vi "GenerateIncrementalBuildInfo.vi"(8 "error in (no error)":errorcluster, 9 "Generated file":T1, 11 "SolutionBuilder in":refnum<class "SolutionBuilder.lvclass">) -> (0 "error out":errorcluster, 3 "SolutionBuilder out":refnum<class "SolutionBuilder.lvclass">)   [LabVIEW 2019, in "SolutionBuilder.lvlib" / "SolutionBuilder.lvclass"]
uses:
  SolutionBuilder.lvclass
  BuildManager/GeneratedFile.ctl
  SolutionBuilder.lvclass/SolutionBuilder.ctl
  Private/IncrementalFileInfoHash.ctl
  Community/SolutionProjectInfo.ctl
  BuildManager/BuildManager.lvclass
  BuildManager/BuildProjectInfo.ctl
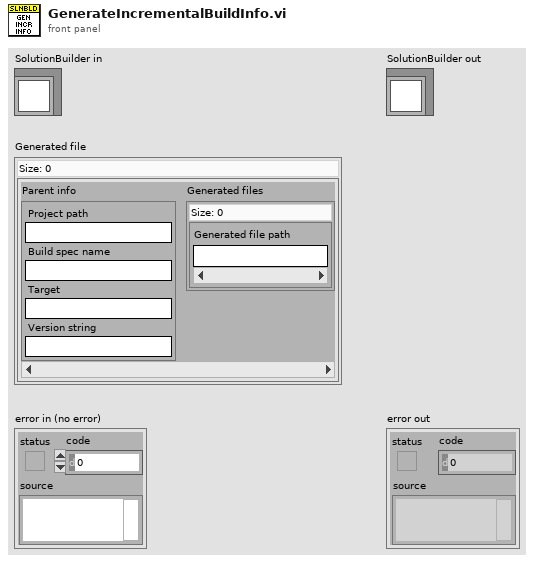
[diagram p1: front panel]
types:
  T1 = typedef "SolutionBuilder.lvlib/BuildManager.lvclass/GeneratedFile.ctl" = map{T2, set{string}}
  T2 = typedef "SolutionBuilder.lvlib/BuildManager.lvclass/BuildProjectInfo.ctl" = cluster{"Project path":string, "Build spec name":string, "Target":string, "Version string":string}
  T3 = typedef "SolutionBuilder.lvlib/SolutionBuilder.lvclass/HashMap.ctl" = map{T4, map{string, string}}
  T4 = typedef "SolutionBuilder.lvlib/SolutionBuilder.lvclass/SolutionProjectInfo.ctl" = cluster{"Project path":string, "Build spec name":string, "Target":string}
  T5 = typedef "SolutionBuilder.lvlib/SolutionBuilder.lvclass/IncrementalFileInfoHash.ctl" = cluster{"Project path":string, "Build spec name":string, "Target":string, "File":string, "MD5 hash":string}
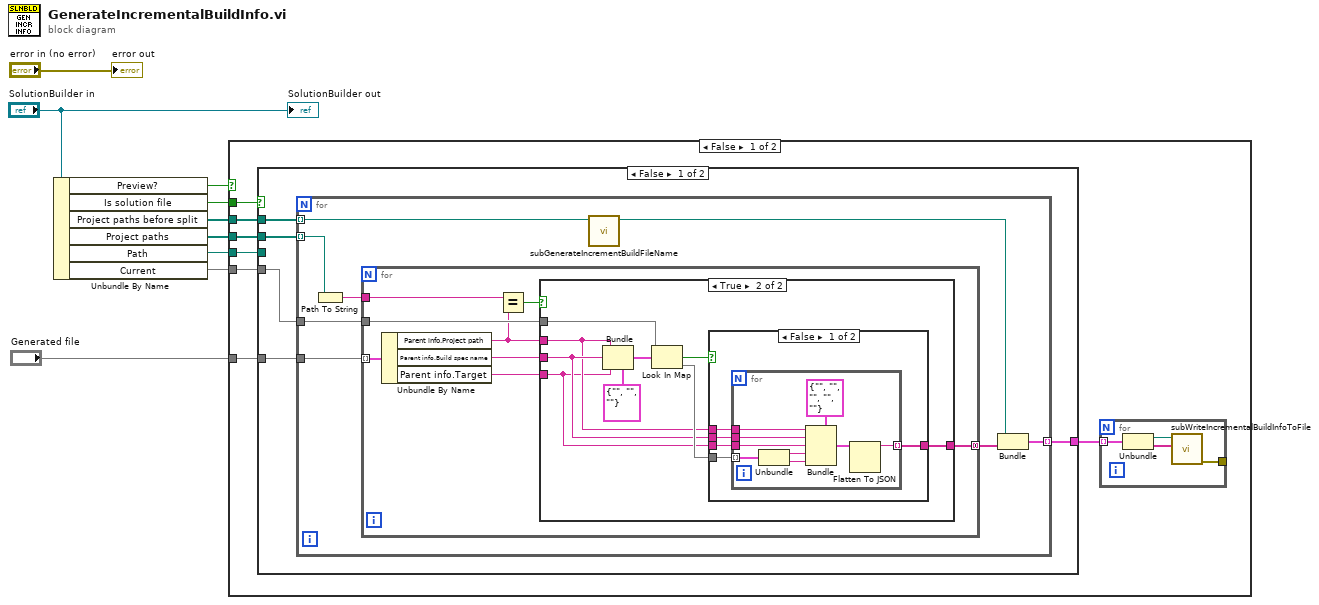
[diagram p0: block diagram]
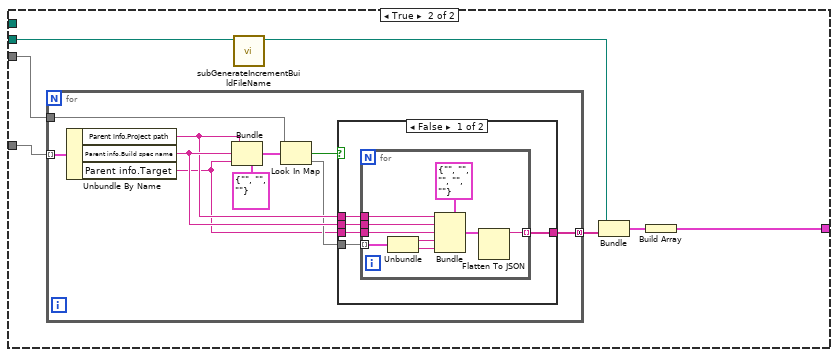
[diagram p4: hidden frame]
diagram:
  n1 = Unbundle By Name("SolutionBuilder in") -> ("Preview?"=w2:bool, "Is solution file"=w3:bool, "Project paths before split"=w8:path[], "Project paths"=w1:path[], "Path"=w7:path, "Current"=w4:T3)
  n2 = case shown="False" w2 {
    tunnel: w8 -> [w16 _]
    tunnel: w7 -> [w15 _]
    tunnel: "Generated file" -> [w14 _]
    tunnel: w4 -> [w13 _]
    tunnel: w3 -> [w12 _]
    tunnel: w1 -> [w10 _]
    frame False {
      n3 = case shown="False" w12 {
        tunnel: w15 -> [_ w67]
        tunnel: [w18 w66] -> w11
        tunnel: w16 -> [w21 _]
        tunnel: w14 -> [w20 w63]
        tunnel: w13 -> [w19 w62]
        tunnel: w10 -> [w17 _]
        frame False {
          n4 = for {
            tunnel: w21 -> [w28] mode=indexing
            tunnel: w19 -> [w26]
            tunnel: w20 -> [w29]
            tunnel: [w24] -> w18 mode=indexing
            tunnel: w17 -> [w22] mode=indexing
            n5 = Path To String(path=w22) -> (string=w27:string)
            n6 = for {
              tunnel: w29 -> [w37] mode=indexing
              tunnel: w27 -> [w33]
              tunnel: w26 -> [w34]
              tunnel: [w36] -> w23 mode=concatenating
              n7 = Unbundle By Name(w37) -> ("Parent info.Project path"=w32:string, "Parent info.Build spec name"=w35:string, "Parent info.Target"=w30:string)
              n8 = Equal?(x=w33, y=w32) -> (x = y?=w31:bool)
              n9 = case shown="True" w31 {
                tunnel: [_ w46] -> w36
                tunnel: w35 -> [_ w40]
                tunnel: w34 -> [_ w44]
                tunnel: w32 -> [_ w39]
                tunnel: w30 -> [_ w38]
                frame False {
                }
                frame True {
                  n10 = Bundle(cluster=T4 {"Project path"="", "Build spec name"="", "Target"=""}, "Project path"=w39, "Build spec name"=w40, "Target"=w38) -> (w42:T4)
                  n11 = Look In Map(map=w44, key=w42) -> (key not found?=w43:bool, value=w41:map{string, string})  [unwired: 1 in]
                  n12 = case shown="False" w43 {
                    tunnel: [w51 _] -> w46
                    tunnel: w41 -> [w50 _]
                    tunnel: w40 -> [w49 _]
                    tunnel: w39 -> [w48 _]
                    tunnel: w38 -> [w47 _]
                    frame False {
                      n13 = for {
                        tunnel: [w59] -> w51 mode=indexing
                        tunnel: w50 -> [w57] mode=indexing
                        tunnel: w49 -> [w56]
                        tunnel: w48 -> [w55]
                        tunnel: w47 -> [w52]
                        n14 = Unbundle(w57) -> ("File"=w53:string, "MD5 hash"=w54:string)
                        n15 = Bundle(cluster=T5 {"Project path"="", "Build spec name"="", "Target"="", "File"="", "MD5 hash"=""}, "Project path"=w55, "Build spec name"=w56, "Target"=w52, "File"=w53, "MD5 hash"=w54) -> (w60:T5)
                        n16 = Flatten To JSON(anything=w60) -> (JSON string=w59:string)  [unwired: 2 in, 1 out]
                      }
                    }
                    frame True {
                    }
                  }
                }
              }
            }
            n17 = call "subGenerateIncrementBuildFileName.vi"("Path in"=w28) -> ("Path out"=w25:path)  [unwired: 10 in]
            n18 = Bundle("Path out"=w25, w23) -> (w24:cluster{"Path out":path, string[]})  [unwired: 1 in]
          }
        }
        frame True {
          n19 = for {
            tunnel: w63 -> [w77] mode=indexing
            tunnel: w62 -> [w74]
            tunnel: [w76] -> w61 mode=concatenating
            n20 = Unbundle By Name(w77) -> ("Parent info.Project path"=w73:string, "Parent info.Build spec name"=w75:string, "Parent info.Target"=w68:string)
            n21 = Bundle(cluster=T4 {"Project path"="", "Build spec name"="", "Target"=""}, "Project path"=w73, "Build spec name"=w75, "Target"=w68) -> (w70:T4)
            n22 = Look In Map(map=w74, key=w70) -> (key not found?=w71:bool, value=w69:map{string, string})  [unwired: 1 in]
            n23 = case shown="False" w71 {
              tunnel: [w82 _] -> w76
              tunnel: w69 -> [w81 _]
              tunnel: w75 -> [w80 _]
              tunnel: w73 -> [w79 _]
              tunnel: w68 -> [w78 _]
              frame False {
                n24 = for {
                  tunnel: [w90] -> w82 mode=indexing
                  tunnel: w81 -> [w88] mode=indexing
                  tunnel: w80 -> [w87]
                  tunnel: w79 -> [w86]
                  tunnel: w78 -> [w83]
                  n25 = Unbundle(w88) -> ("File"=w84:string, "MD5 hash"=w85:string)
                  n26 = Bundle(cluster=T5 {"Project path"="", "Build spec name"="", "Target"="", "File"="", "MD5 hash"=""}, "Project path"=w86, "Build spec name"=w87, "Target"=w83, "File"=w84, "MD5 hash"=w85) -> (w91:T5)
                  n27 = Flatten To JSON(anything=w91) -> (JSON string=w90:string)  [unwired: 2 in, 1 out]
                }
              }
              frame True {
              }
            }
          }
          n28 = call "subGenerateIncrementBuildFileName.vi"("Path in"=w67) -> ("Path out"=w65:path)  [unwired: 10 in]
          n29 = Bundle("Path out"=w65, w61) -> (w64:cluster{"Path out":path, string[]})  [unwired: 1 in]
          n30 = Build Array(w64) -> (w66:cluster{"Path out":path, string[]}[])
        }
      }
      n31 = for {
        tunnel: w11 -> [w95] mode=indexing
        tunnel: [w92] -> _
        n32 = Unbundle(w95) -> ("Path out"=w94:path, w93:string[])
        n33 = call "subWriteIncrementalBuildInfoToFile.vi"("Files"=w93, "Path in"=w94) -> ("error out"=w92:errorcluster)  [unwired: 9 in]
      }
    }
    frame True {
    }
  }
  "error out" <- "error in (no error)"
  "SolutionBuilder out" <- "SolutionBuilder in"
